vi "GetWyPts_CmdNum.vi"(8 "error in (no error)":errorcluster, 10 "CmdNum":i32) -> (0 "error out":errorcluster, 1 "found":bool, 2 "WyPts":string[](array[string]))   [LabVIEW 2020, in "WyPtDict.lvlib"]
doc: "Developed by Kevin Thompson\nkevin@thompsonengineering.net\n\nCopyright 2021\nThompson Engineering, LLC"
uses:
  WyPtDict.lvlib
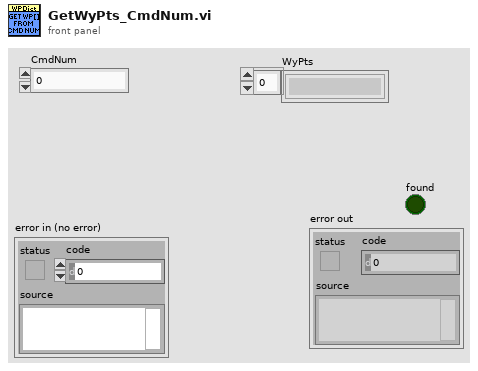
[diagram p1: front panel]
types:
  T1 = typedef "TD Dynamic CVT DVR--ref.ctl" = refnum<data-value>
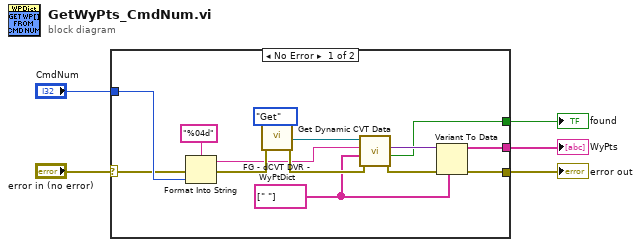
[diagram p0: block diagram]
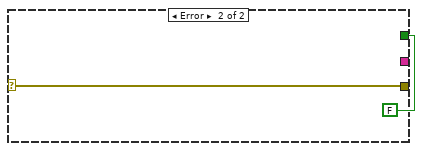
[diagram p2: hidden frame]
diagram:
  n1 = case shown="No Error" "error in (no error)" {
    selector: "error in (no error)" -> [w8 w21]
    tunnel: [w13 w21] -> w5
    tunnel: "CmdNum" -> [w10 _]
    tunnel: [w14 _] -> w2
    tunnel: [w12 FALSE ("found")] -> w1
    frame No Error {
      w11 = string[] [" "]
      n2 = Format Into String(format string="%04d", error in=w8, w10) -> (resulting string=w6:string, error out=w7:errorcluster)  [unwired: 1 in]
      n3 = call "FG - dCVT DVR - WyPtDict.vi"("error in (no error)"=w7, "Action (Get)"=enum16{"Init", "Get", "Set"}."Get") -> ("dCVT WyPt out"=w18:T1, "error out"=w17:errorcluster)  [unwired: 7 in]
      n4 = call <vilib>:"Get Dynamic CVT Data.vi"("error in (no error)"=w17, "default value (empty variant)"=w11, "DataName"=w6, "dCVT DVR"=w18) -> ("error out"=w16:errorcluster, "found"=w12:bool, "value"=w15:variant)  [unwired: 4 in, 1 out]
      n5 = Variant To Data(error in=w16, type=w11, Variant=w15) -> (data=w14:string[], error out=w13:errorcluster)
    }
    frame Error {
    }
  }
  "error out" <- w5
  "WyPts" <- w2
  "found" <- w1
